vi "read_PulseDelay_subvi.vi"(8 "error in (no error)":errorcluster, 9 "Address (0x50) in":u16=80 max=1023 format="%.0x", 10 "Num Bytes to Fetch (64) in":u8=64 min=1, 11 "Aardvark Handle":i32 min=0) -> (0 "error out":errorcluster, 3 "PulseDelay":dbl)   [LabVIEW 2014]
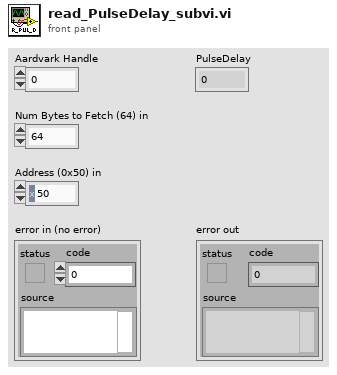
[diagram p1: front panel]
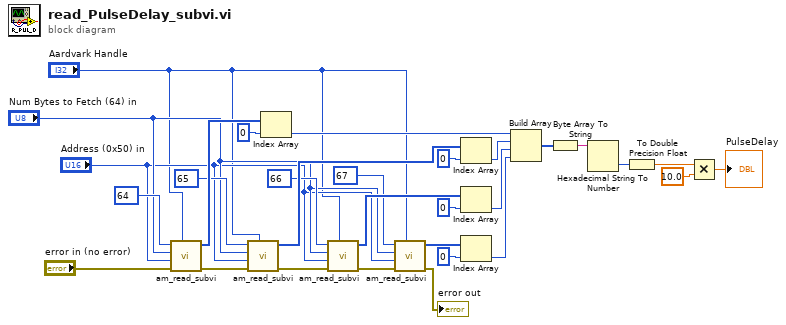
[diagram p0: block diagram]
diagram:
  n1 = call "am_read_subvi.vi"("Aardvark Handle in"="Aardvark Handle", "error in (no error)"="error in (no error)", "Address (0x50) in"="Address (0x50) in", "Num Bytes to Fetch (64)"="Num Bytes to Fetch (64) in", "Memory ADD"=u16 64) -> ("error out"=w2:errorcluster, "Array"=w14:u8[])  [unwired: 5 in]
  n2 = call "am_read_subvi.vi"("Aardvark Handle in"="Aardvark Handle", "error in (no error)"=w2, "Address (0x50) in"="Address (0x50) in", "Num Bytes to Fetch (64)"="Num Bytes to Fetch (64) in", "Memory ADD"=u16 65) -> ("error out"=w3:errorcluster, "Array"=w18:u8[])  [unwired: 5 in]
  n3 = Index Array(array=w14, index=0) -> (element=w21:u8)
  n4 = call "am_read_subvi.vi"("Aardvark Handle in"="Aardvark Handle", "error in (no error)"=w3, "Address (0x50) in"="Address (0x50) in", "Num Bytes to Fetch (64)"="Num Bytes to Fetch (64) in", "Memory ADD"=u16 66) -> ("error out"=w4:errorcluster, "Array"=w19:u8[])  [unwired: 5 in]
  n5 = call "am_read_subvi.vi"("Aardvark Handle in"="Aardvark Handle", "error in (no error)"=w4, "Address (0x50) in"="Address (0x50) in", "Num Bytes to Fetch (64)"="Num Bytes to Fetch (64) in", "Memory ADD"=u16 67) -> ("error out"=→"error out":errorcluster, "Array"=w20:u8[])  [unwired: 5 in]
  n6 = Index Array(array=w18, index=0) -> (element=w22:u8)
  n7 = Index Array(array=w19, index=0) -> (element=w23:u8)
  n8 = Index Array(array=w20, index=0) -> (element=w24:u8)
  n9 = Build Array(w21, w22, w23, w24) -> (w26:u8[])
  n10 = Byte Array To String(unsigned byte array=w26) -> (string=w27:string)
  n11 = Hexadecimal String To Number(string=w27) -> (number=w29:u32)  [unwired: 2 in, 1 out]
  n12 = To Double Precision Float(number=w29) -> (double precision float=w30:dbl)
  n13 = Multiply(x=w30, y=10.0) -> (x*y=→"PulseDelay":dbl)
